vi "MaquinaDeEstados.vi"() -> ()   [LabVIEW 2022 SP3]
panel:
  out "Current State":string
  in  "C":bool
  in  "B":bool
  in  "A":bool
  in  "stop":bool
  # "Máquinas de Estado"
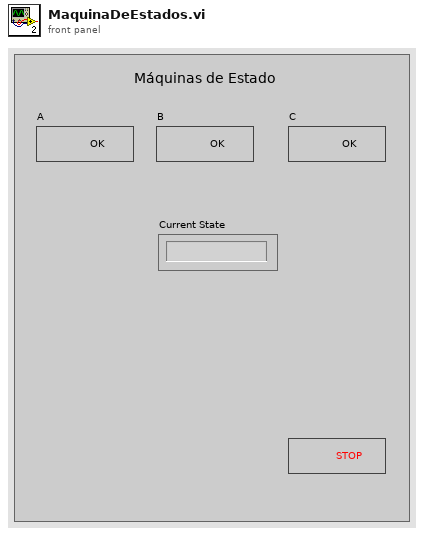
[diagram p1: front panel]
types:
  T1 = enum16{"Start", "State 1", "State 2", "State 3", "State 4", "End"}
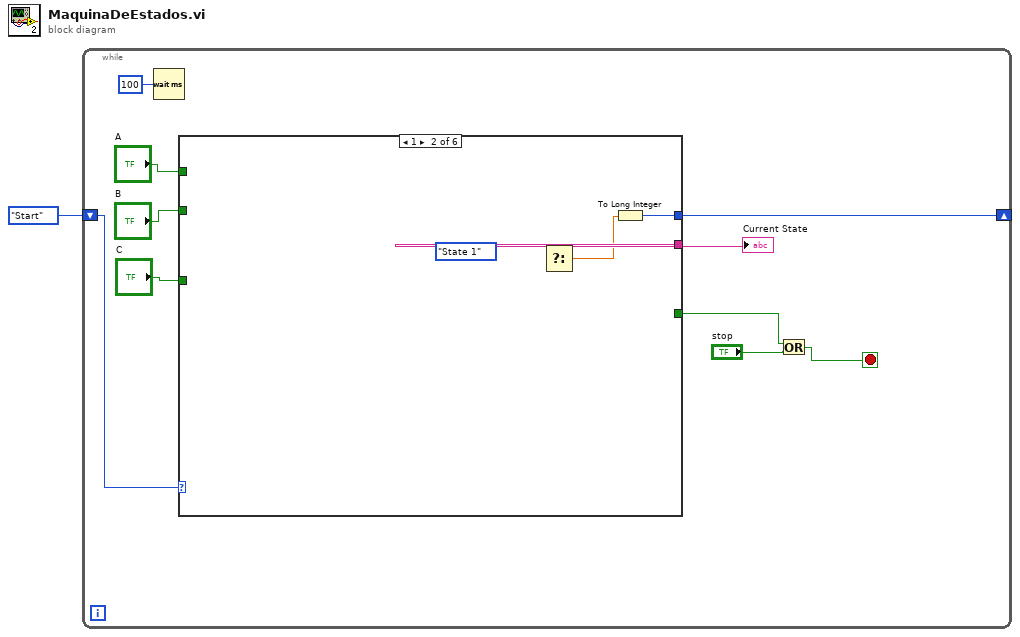
[diagram p0: block diagram]
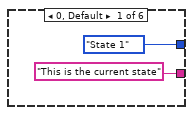
[diagram p2: hidden frame]
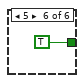
[diagram p6: hidden frame]
diagram:
  n1 = while {
    shift-right: [w6] -> _
    shift-left: T1."Start" -> [w5]
    stop <- w2 stop-if-true
    n2 = Wait (ms)(milliseconds to wait=u32 100) -> ()  [unwired: 1 out]
    n3 = case shown="1" w5 {
      tunnel: [T1."State 1" w15 _ _ _ _] -> w6
      tunnel: ["This is the current state" _ _ _ _ _] -> w10
      tunnel: "A" -> [_ _ _ _ _ _]
      tunnel: "C" -> [_ _ _ _ _ _]
      tunnel: "B" -> [_ _ _ _ _ _]
      tunnel: [_ _ _ _ _ TRUE] -> w4
      frame 0, Default {
      }
      frame 1 {
        (unwired) T1."State 1"
        n4 = Select() -> (s? t:f=w14:dbl)  [unwired: 3 in]
        n5 = To Long Integer(number=w14) -> (32bit integer=w15:i32)
      }
      frame 2 {
      }
      frame 3 {
      }
      frame 4 {
      }
      frame 5 {
      }
    }
    "Current State" <- w10
    n6 = Or(x=w4, y="stop") -> (x .or. y?=w2:bool)
  }
